vi "Hit Detect.vi"(7 "Visible only? [T]":bool=TRUE, 8 "error in (no error)":errorcluster, 10 "Coords":T1, 11 "IContainer in":refnum<class "IContainer.lvclass">) -> (0 "error out":errorcluster, 1 "Hit?":bool, 2 "In Object":string[](array[string]), 3 "IContainer out":refnum<class "IContainer.lvclass">)   [LabVIEW 2013, in "IContainer.lvclass"]
doc: "Copyright 2018, Wiebe Walstra, wiebe@carya.nl."
uses:
  IContainer.lvclass
  <vilib>/Utility/miscctls.llb/LVPoint32TypeDef.ctl
  IObject.lvclass
  IContainer.lvclass/IContainer.ctl
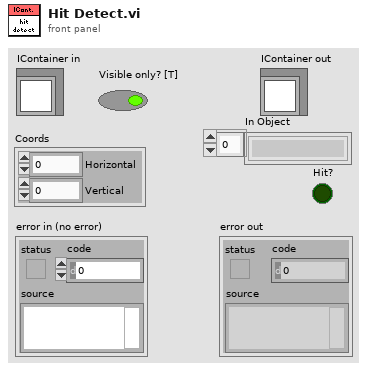
[diagram p1: front panel]
types:
  T1 = typedef "LVPoint32TypeDef.ctl" = cluster{"Horizontal":i32, "Vertical":i32}
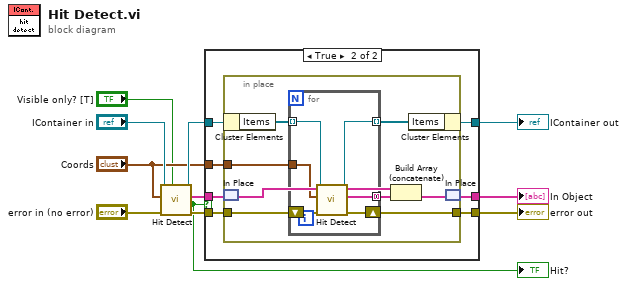
[diagram p0: block diagram]
diagram:
  n1 = call-parent "Hit Detect.vi"("Visible only? [T]"="Visible only? [T]", "error in (no error)"="error in (no error)", "Coords"="Coords", "IObject in"="IContainer in") -> ("error out"=w9:errorcluster, "Hit?"=w2:bool, "In Object"=w3:string[], "IObject out"=w7:refnum<class "IContainer.lvclass">)  [unwired: 4 in]
  "Hit?" <- w2
  n2 = case shown="True" w2 {
    tunnel: [w14 w21] -> w11
    tunnel: w9 -> [w14 w20]
    tunnel: w7 -> [w13 w18]
    tunnel: "Coords" -> [_ w19]
    tunnel: [w13 w17] -> w6
    tunnel: w3 -> [w12 w16]
    tunnel: [w12 w15] -> w1
    frame False {
    }
    frame True {
      n3 = in-place {
        in-place-border: [w29] -> w21
        in-place-border: w20 -> [w28]
        in-place-border: w19 -> [w27]
        n4 = in-place-cluster #1(w18) -> ("Items"=w26:refnum<class "IObject.lvclass">[])
        n5 = in-place-match #2(w16) -> (w23:string[])
        n6 = for {
          tunnel: w27 -> [w33]
          shift-right: [w35] -> w29
          shift-left: w28 -> [w34]
          tunnel: w26 -> [w32] mode=indexing
          tunnel: [w31] -> w25 mode=indexing
          tunnel: [w30] -> w24 mode=concatenating
          n7 = call-dynamic "Hit Detect.vi"("error in (no error)"=w34, "Coords"=w33, "IObject in"=w32) -> ("error out"=w35:errorcluster, "In Object"=w30:string[], "IObject out"=w31:refnum<class "IObject.lvclass">)  [unwired: 5 in, 1 out]
        }
        n8 = Build Array (concatenate)(w23, w24) -> (w22:string[])
        n9 = in-place-cluster #1("Items"=w25) -> (w17:refnum<class "IContainer.lvclass">)
        n10 = in-place-match #2(w22) -> (w15:string[])
      }
    }
  }
  "error out" <- w11
  "IContainer out" <- w6
  "In Object" <- w1
